vi "Travel the Board Following Map Steps.vi"(4 "Start Location":T2, 5 "Steps":T3[](array[typedef]), 7 "Facing Direction in":T1, 9 "Board Map":T5[][](array[typedef]) items=["Empty", "Portal", "Open", "Wall", ">", "<", ">-^", ">-v", "^-<", "v-<"]) -> (0 "Last Location":T2, 1 "Facing Direction out":T1, 3 "Board Travel":T5[][][](array[typedef]) items=["Empty", "Portal", "Open", "Wall", ">", "<", ">-^", ">-v", "^-<", "v-<"])   [LabVIEW 2020, in "AoC 2022.lvlib"]
uses:
  AoC 2022.lvlib
  Day 15 - Beacon Exclusion Zone/private/Location.ctl
  Map Tile.ctl
  Map Action Step.ctl
  Map Action.ctl
  Map Direction.ctl
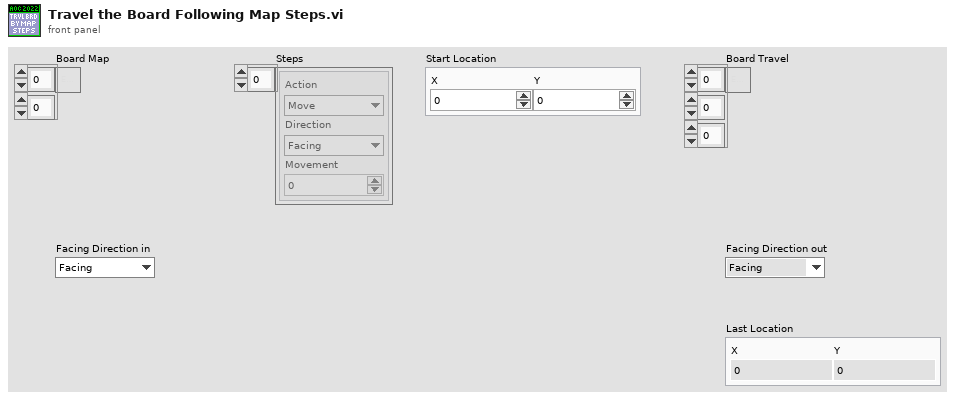
[diagram p1: front panel]
types:
  T1 = typedef "AoC 2022.lvlib/Map Direction.ctl" = enum16{"Facing", "Right", "Left", "Up", "Down"}
  T2 = typedef "AoC 2022.lvlib/Location.ctl" = cluster{"X":i32, "Y":i32}
  T3 = typedef "AoC 2022.lvlib/Map Action Step.ctl" = cluster{"Action":T4, "Direction":T1, "Movement":i32}
  T4 = typedef "AoC 2022.lvlib/Map Action.ctl" = enum16{"Move", "Turn"}
  T5 = typedef "AoC 2022.lvlib/Map Tile.ctl" = u16
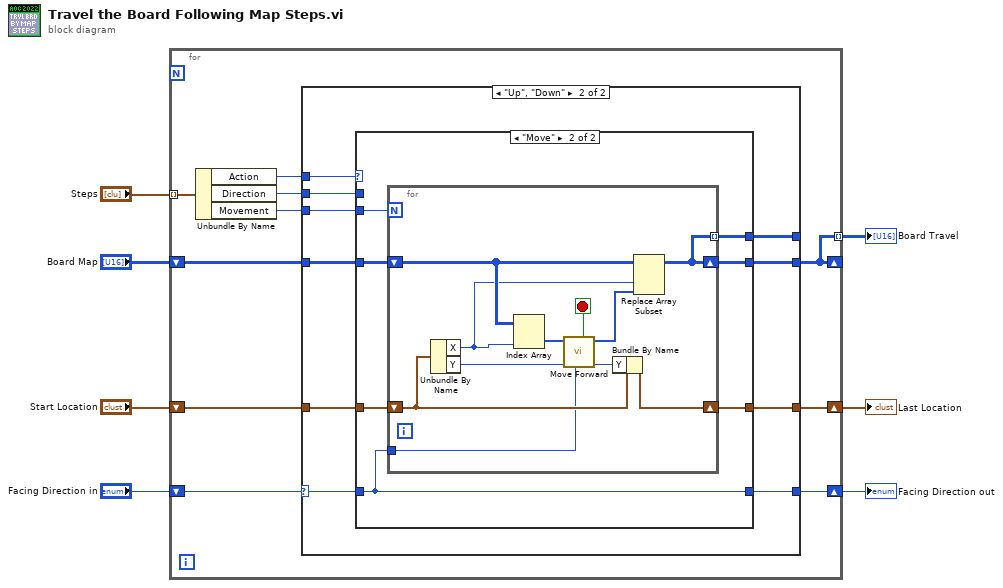
[diagram p0: block diagram]
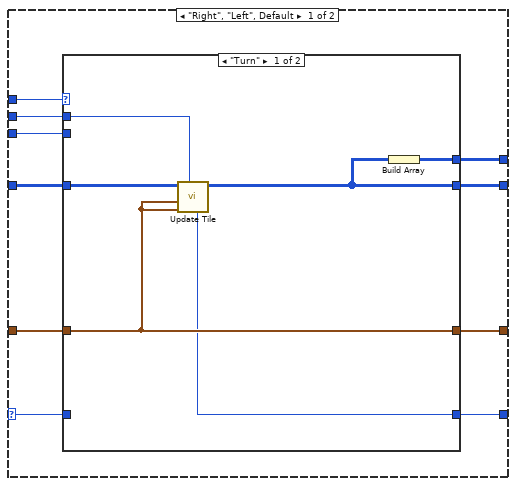
[diagram p2: hidden frame]
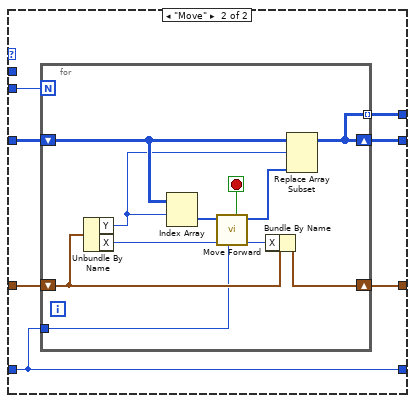
[diagram p3: hidden frame]
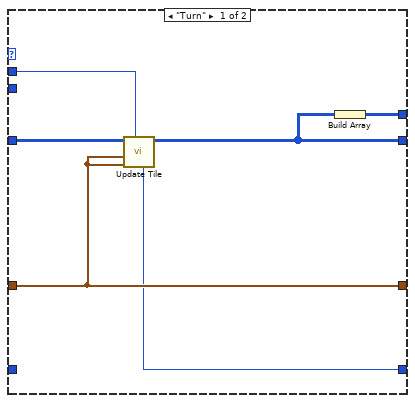
[diagram p4: hidden frame]
diagram:
  n1 = for {
    tunnel: "Steps" -> [w17] mode=indexing
    shift-right: [w8] -> _
    shift-left: "Board Map" -> [w16]
    tunnel: [w8] -> w5 mode=indexing
    shift-right: [w14] -> w2
    shift-left: "Start Location" -> [w15]
    shift-right: [w13] -> w3
    shift-left: "Facing Direction in" -> [w12]
    n2 = Unbundle By Name(w17) -> ("Action"=w11:T4, "Direction"=w10:T1, "Movement"=w9:i32)
    n3 = case shown="\"Up\", \"Down\"" w12 {
      selector: w12 -> [w21 w55]
      tunnel: [w19 w53] -> w8
      tunnel: w16 -> [w27 w61]
      tunnel: w15 -> [w26 w60]
      tunnel: [w24 w58] -> w14
      tunnel: [w20 w54] -> w13
      tunnel: w11 -> [w23 w57]
      tunnel: w10 -> [w22 w56]
      tunnel: w9 -> [w25 w59]
      tunnel: [w18 w52] -> _
      frame "Right", "Left", Default {
        n4 = case shown="\"Turn\"" w23 {
          tunnel: w27 -> [w33 w38]
          tunnel: w26 -> [w32 w40]
          tunnel: w25 -> [_ w36]
          tunnel: [w32 w39] -> w24
          tunnel: w22 -> [w31 _]
          tunnel: w21 -> [_ w34]
          tunnel: [w30 w34] -> w20
          tunnel: [w29 w37] -> w19
          tunnel: [w28 w35] -> w18
          frame "Turn" {
            n5 = call "Update Tile.vi"("Turn Direction"=w31, "Current Location"=w32, "Next Location"=w32, "Board Map in"=w33) -> ("Board Map out"=w29:T5[][], "Next Direction"=w30:T1)  [unwired: 4 in]
            n6 = Build Array(w29) -> (w28:T5[][][])
          }
          frame "Move" {
            n7 = for {
              N: w36 -> [_]
              shift-right: [w48] -> w39
              shift-left: w40 -> [w51]
              shift-right: [w43] -> w37
              shift-left: w38 -> [w46]
              tunnel: [w43] -> w35 mode=indexing
              tunnel: w34 -> [w41]
              stop <- w42 stop-if-true
              n8 = Unbundle By Name(w51) -> ("Y"=w45:i32, "X"=w49:i32)
              n9 = Index Array(array=w46, index (row)=w45) -> (element=w50:T5[])  [unwired: 1 in]
              n10 = call "Move Forward.vi"("Facing Direction"=w41, "Current Position"=w49, "Facing Road in"=w50) -> ("Next Position"=w47:i32, "Facing Road out"=w44:T5[], "Hit the Wall ?"=w42:bool)  [unwired: 4 in]
              n11 = Bundle By Name(cluster=w51, "X"=w47) -> (w48:T2)
              n12 = Replace Array Subset(array=w46, new element=w44, index (row)=w45) -> (w43:T5[][])  [unwired: 1 in]
            }
          }
        }
      }
      frame "Up", "Down" {
        n13 = case shown="\"Move\"" w57 {
          tunnel: w61 -> [w67 w72]
          tunnel: w60 -> [w66 w74]
          tunnel: w59 -> [_ w70]
          tunnel: [w66 w73] -> w58
          tunnel: w56 -> [w65 _]
          tunnel: w55 -> [_ w68]
          tunnel: [w64 w68] -> w54
          tunnel: [w63 w71] -> w53
          tunnel: [w62 w69] -> w52
          frame "Turn" {
            n14 = call "Update Tile.vi"("Turn Direction"=w65, "Current Location"=w66, "Next Location"=w66, "Board Map in"=w67) -> ("Board Map out"=w63:T5[][], "Next Direction"=w64:T1)  [unwired: 4 in]
            n15 = Build Array(w63) -> (w62:T5[][][])
          }
          frame "Move" {
            n16 = for {
              N: w70 -> [_]
              shift-right: [w82] -> w73
              shift-left: w74 -> [w85]
              shift-right: [w78] -> w71
              shift-left: w72 -> [w80]
              tunnel: [w78] -> w69 mode=indexing
              tunnel: w68 -> [w76]
              stop <- w77 stop-if-true
              n17 = Unbundle By Name(w85) -> ("X"=w75:i32, "Y"=w83:i32)
              n18 = Index Array(array=w80, index (col)=w75) -> (element=w84:T5[])  [unwired: 1 in]
              n19 = call "Move Forward.vi"("Facing Direction"=w76, "Current Position"=w83, "Facing Road in"=w84) -> ("Next Position"=w81:i32, "Facing Road out"=w79:T5[], "Hit the Wall ?"=w77:bool)  [unwired: 4 in]
              n20 = Bundle By Name(cluster=w85, "Y"=w81) -> (w82:T2)
              n21 = Replace Array Subset(array=w80, new element=w79, index (col)=w75) -> (w78:T5[][])  [unwired: 1 in]
            }
          }
        }
      }
    }
  }
  "Board Travel" <- w5
  "Facing Direction out" <- w3
  "Last Location" <- w2
